vi "Controller Settings FG.vi"(7 "Action":T2, 8 "error in (no error)":errorcluster, 10 "Controller Settings":T3={"Output Max"=100.0, "Output Min"=0.0, "Setpoint Max"=100.0, "Setpoint Min"=0.0, "Use External Setpoint"=FALSE, "Output Rate Limiter"=10.0}, 11 "Node Ptr":T1 format="%.0x") -> (0 "error out":errorcluster, 2 "Controller Settings":T3, 3 "Item Ref out":T1=18446744073709551615 format="%.0x")   [LabVIEW 2019, in "Control Addon System Explorer.lvlib"]
uses:
  Control Addon System Explorer.lvlib
  <vilib>/NI VeriStand/Custom Device API/Custom Device Item Ref.ctl
  Addon Shared/Types/Controller Settings.ctl
  Types/Action.ctl
  Addon Shared/SubVIs/Constants.vi
  <vilib>/NI VeriStand/Custom Device API/Get Item Property (Double).vi
  <vilib>/NI VeriStand/Custom Device API/Get Item Property (Boolean).vi
  <vilib>/NI VeriStand/Custom Device API/Set Item Property (Double).vi
  <vilib>/NI VeriStand/Custom Device API/Set Item Property (Boolean).vi
  <vilib>/NI VeriStand/Custom Device API/Custom Device API.lvlib
  Addon Shared/Control Addon Shared.lvlib
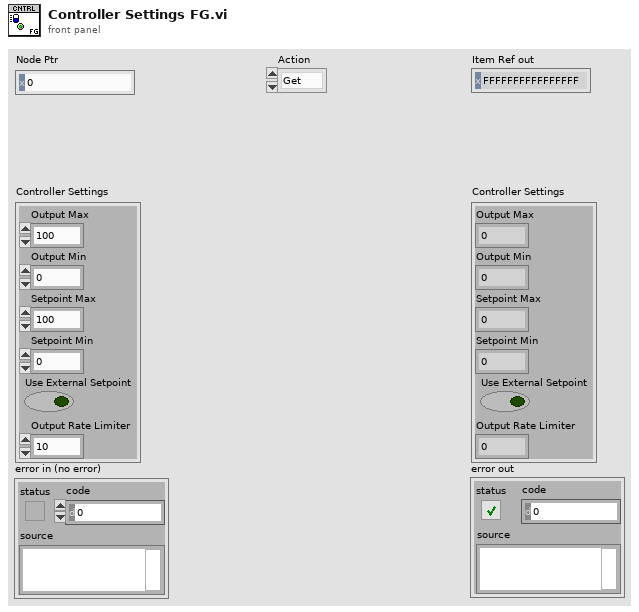
[diagram p1: front panel]
types:
  T1 = typedef "Custom Device API.lvlib/Custom Device Item Ref.ctl" = u64
  T2 = typedef "Control Addon System Explorer.lvlib/Action.ctl" = enum16{"Get", "Set"}
  T3 = typedef "Control Addon Shared.lvlib/Controller Settings.ctl" = cluster{"Output Max":dbl, "Output Min":dbl, "Setpoint Max":dbl, "Setpoint Min":dbl, "Use External Setpoint":bool, "Output Rate Limiter":dbl}
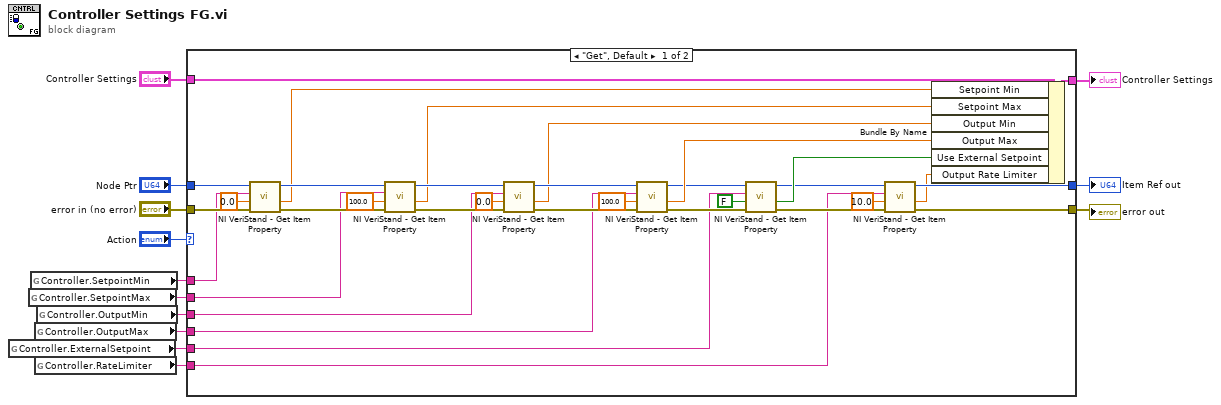
[diagram p0: block diagram]
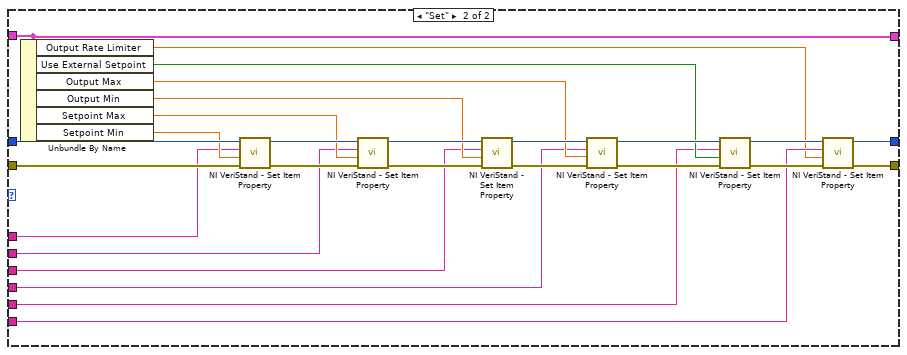
[diagram p2: hidden frame]
diagram:
  n1 = global read "Constants.vi" "Controller.ExternalSetpoint"() -> (w2:string)
  n2 = global read "Constants.vi" "Controller.SetpointMax"() -> (w5:string)
  n3 = global read "Constants.vi" "Controller.SetpointMin"() -> (w6:string)
  n4 = global read "Constants.vi" "Controller.OutputMax"() -> (w3:string)
  n5 = global read "Constants.vi" "Controller.RateLimiter"() -> (w1:string)
  n6 = global read "Constants.vi" "Controller.OutputMin"() -> (w4:string)
  n7 = case shown="\"Get\", Default" "Action" {
    tunnel: "Node Ptr" -> [w34 w74]
    tunnel: "error in (no error)" -> [w41 w73]
    tunnel: "Controller Settings" -> [w47 w59]
    tunnel: [w46 w59] -> w9
    tunnel: [w19 w51] -> w7
    tunnel: [w17 w50] -> w8
    tunnel: w6 -> [w33 w58]
    tunnel: w5 -> [w32 w57]
    tunnel: w4 -> [w31 w56]
    tunnel: w3 -> [w30 w55]
    tunnel: w2 -> [w29 w54]
    tunnel: w1 -> [w16 w49]
    frame "Get", Default {
      n8 = call-poly <vilib>:"NI VeriStand - Get Item Property.vi"("error in (no error)"=w41, "Default Value"=0.0, "Property Name"=w33, "Item Ref in"=w34) -> ("error out"=w45:errorcluster, "Value"=w28:dbl, "Item Ref out"=w35:T1)  [unwired: 4 in, 1 out]
      n9 = call-poly <vilib>:"NI VeriStand - Get Item Property.vi"("error in (no error)"=w45, "Default Value"=100.0, "Property Name"=w32, "Item Ref in"=w35) -> ("error out"=w44:errorcluster, "Value"=w27:dbl, "Item Ref out"=w36:T1)  [unwired: 4 in, 1 out]
      n10 = call-poly <vilib>:"NI VeriStand - Get Item Property.vi"("error in (no error)"=w44, "Default Value"=0.0, "Property Name"=w31, "Item Ref in"=w36) -> ("error out"=w43:errorcluster, "Value"=w26:dbl, "Item Ref out"=w37:T1)  [unwired: 4 in, 1 out]
      n11 = call-poly <vilib>:"NI VeriStand - Get Item Property.vi"("error in (no error)"=w43, "Default Value"=100.0, "Property Name"=w30, "Item Ref in"=w37) -> ("error out"=w42:errorcluster, "Value"=w39:dbl, "Item Ref out"=w38:T1)  [unwired: 4 in, 1 out]
      n12 = call-poly <vilib>:"NI VeriStand - Get Item Property.vi"("error in (no error)"=w42, "Default Value"=FALSE, "Property Name"=w29, "Item Ref in"=w38) -> ("error out"=w20:errorcluster, "Value"=w40:bool, "Item Ref out"=w18:T1)  [unwired: 4 in, 1 out]
      n13 = call-poly <vilib>:"NI VeriStand - Get Item Property.vi"("error in (no error)"=w20, "Default Value"=10.0, "Property Name"=w16, "Item Ref in"=w18) -> ("error out"=w19:errorcluster, "Value"=w15:dbl, "Item Ref out"=w17:T1)  [unwired: 4 in, 1 out]
      n14 = Bundle By Name(cluster=w47, "Setpoint Min"=w28, "Setpoint Max"=w27, "Output Min"=w26, "Output Max"=w39, "Use External Setpoint"=w40, "Output Rate Limiter"=w15) -> (w46:T3)
    }
    frame "Set" {
      n15 = Unbundle By Name(w59) -> ("Output Rate Limiter"=w48:dbl, "Use External Setpoint"=w60:bool, "Output Max"=w61:dbl, "Output Min"=w62:dbl, "Setpoint Max"=w63:dbl, "Setpoint Min"=w64:dbl)
      n16 = call-poly <vilib>:"NI VeriStand - Set Item Property.vi"("error in (no error)"=w73, "Value"=w64, "Property Name"=w58, "Item Ref in"=w74) -> ("error out"=w67:errorcluster, "Item Ref out"=w72:T1)  [unwired: 5 in, 1 out]
      n17 = call-poly <vilib>:"NI VeriStand - Set Item Property.vi"("error in (no error)"=w67, "Value"=w63, "Property Name"=w57, "Item Ref in"=w72) -> ("error out"=w68:errorcluster, "Item Ref out"=w71:T1)  [unwired: 5 in, 1 out]
      n18 = call-poly <vilib>:"NI VeriStand - Set Item Property.vi"("error in (no error)"=w68, "Value"=w62, "Property Name"=w56, "Item Ref in"=w71) -> ("error out"=w69:errorcluster, "Item Ref out"=w70:T1)  [unwired: 5 in, 1 out]
      n19 = call-poly <vilib>:"NI VeriStand - Set Item Property.vi"("error in (no error)"=w69, "Value"=w61, "Property Name"=w55, "Item Ref in"=w70) -> ("error out"=w65:errorcluster, "Item Ref out"=w66:T1)  [unwired: 5 in, 1 out]
      n20 = call-poly <vilib>:"NI VeriStand - Set Item Property.vi"("error in (no error)"=w65, "Value"=w60, "Property Name"=w54, "Item Ref in"=w66) -> ("error out"=w52:errorcluster, "Item Ref out"=w53:T1)  [unwired: 5 in, 1 out]
      n21 = call-poly <vilib>:"NI VeriStand - Set Item Property.vi"("error in (no error)"=w52, "Value"=w48, "Property Name"=w49, "Item Ref in"=w53) -> ("error out"=w51:errorcluster, "Item Ref out"=w50:T1)  [unwired: 5 in, 1 out]
    }
  }
  "Controller Settings" <- w9
  "Item Ref out" <- w8
  "error out" <- w7
